vi "Generate Transfer Function.vi"(8 "Error In":errorcluster, 11 "ADC in":refnum<class "ADC.lvclass">) -> (0 "Error Out":errorcluster, 3 "ADC out":refnum<class "ADC.lvclass">)   [LabVIEW 2023, in "ADC.lvclass"]
uses:
  ADC.lvclass
  C:/Git/Ancy-LV-Assignments-TIPS-2/src/Assignment 4/SDLC - DNL and INL Testing/INL and DNL Calculation/Classes/Mode/Mode.lvclass
  Typedef/Transfer Function.ctl
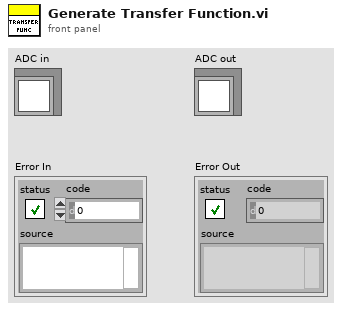
[diagram p1: front panel]
types:
  T1 = typedef "Transfer Function.ctl" = cluster{"Ideal voltage":dbl[], "Digital Code":dbl[]}
  T2 = typedef "Input Voltage Parameters.ctl" = cluster{"Voltage Max":dbl, "Voltage Min":dbl, "No.of bits":dbl}
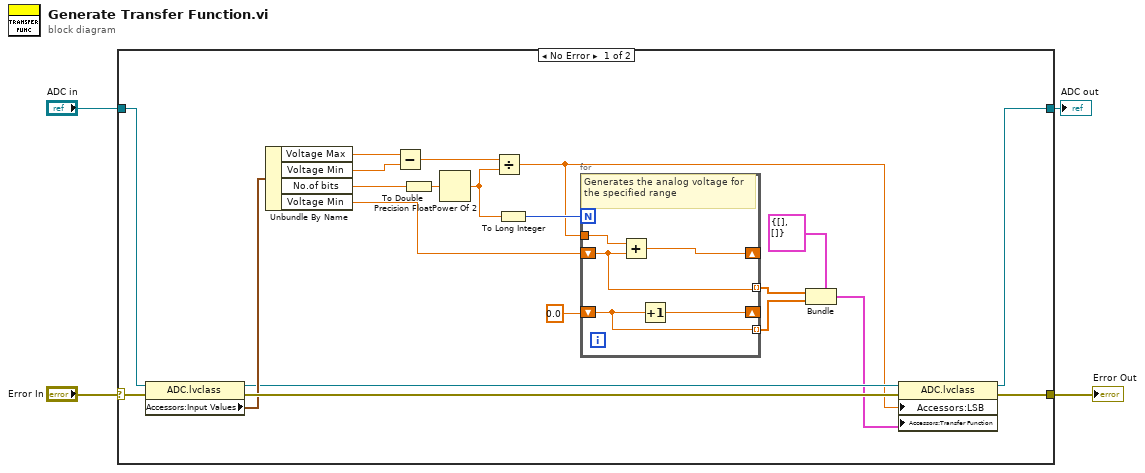
[diagram p0: block diagram]
diagram:
  n1 = case shown="No Error" "Error In" {
    selector: "Error In" -> [w15 w32]
    tunnel: [w10 w32] -> w3
    tunnel: [w5 w31] -> w1
    tunnel: "ADC in" -> [w12 w31]
    frame No Error {
      n2 = property class="ADC.lvclass"(reference=w12, error in=w15) -> (reference out=w9:refnum<class "ADC.lvclass">, error out=w13:errorcluster, "Accessors:Input Values"=w11:T2)
      n3 = Unbundle By Name(w11) -> ("Voltage Max"=w21:dbl, "Voltage Min"=w20:dbl, "No.of bits"=w19:dbl, "Voltage Min"=w18:dbl)
      n4 = Subtract(x=w21, y=w20) -> (x-y=w22:dbl)
      n5 = To Double Precision Float(number=w19) -> (double precision float=w25:dbl)
      n6 = Power Of 2(x=w25) -> (2^x=w24:dbl)
      n7 = Divide(x=w22, y=w24) -> (x/y=w7:dbl)
      n8 = To Long Integer(number=w24) -> (32bit integer=w23:i32)
      n9 = for {
        N: w23 -> [_]
        shift-right: [w30] -> _
        shift-left: w18 -> [w26]
        tunnel: w7 -> [w28]
        tunnel: [w26] -> w14 mode=indexing
        shift-right: [w29] -> _
        shift-left: 0.0 -> [w27]
        tunnel: [w27] -> w6 mode=indexing
        # "Generates the analog voltage for the specified range"
        n10 = Add(x=w28, y=w26) -> (x+y=w30:dbl)
        n11 = Increment(x=w27) -> (x+1=w29:dbl)
      }
      n12 = Bundle(cluster=T1 {"Ideal voltage"=[], "Digital Code"=[]} ("output cluster"), "Ideal voltage"=w14, "Digital Code"=w6) -> (w8:T1)
      n13 = property class="ADC.lvclass"(reference=w9, error in=w13, "Accessors:LSB"=w7, "Accessors:Transfer Function"=w8) -> (reference out=w5:refnum<class "ADC.lvclass">, error out=w10:errorcluster)
    }
    frame Error {
    }
  }
  "Error Out" <- w3
  "ADC out" <- w1
